vi "Hide.vi"(8 "error in (no error)":errorcluster, 10 "Visible":bool, 11 "Array":refnum<vi>[](array[refnum])) -> (0 "error out":errorcluster)   [LabVIEW 2013]
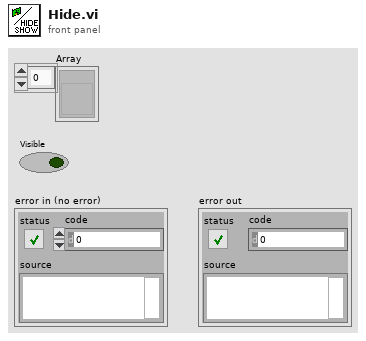
[diagram p1: front panel]
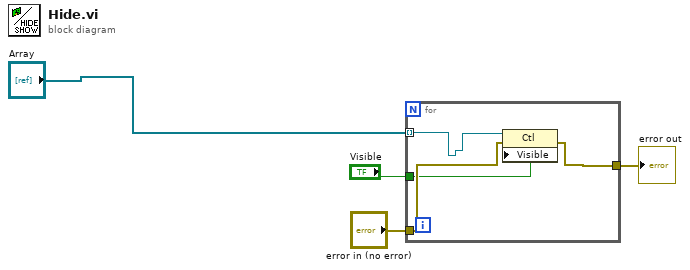
[diagram p0: block diagram]
diagram:
  n1 = for {
    tunnel: "error in (no error)" -> [w7]
    tunnel: [w6] -> w1
    tunnel: "Array" -> [w8] mode=indexing
    tunnel: "Visible" -> [w5]
    n2 = property class="Ctl"(reference=w8, error in=w7, "Visible"=w5) -> (error out=w6:errorcluster)  [unwired: 1 out]
  }
  "error out" <- w1
